vi "ERR HANDLER - Processor Loop.vi"   [LabVIEW 2013]
uses:
  Error Queue Message.ctl
types:
  T1 = typedef "Error Queue Message.ctl" = cluster{"Command":enum16{"HANDLE ERROR", "EXIT"}, "Data":variant}
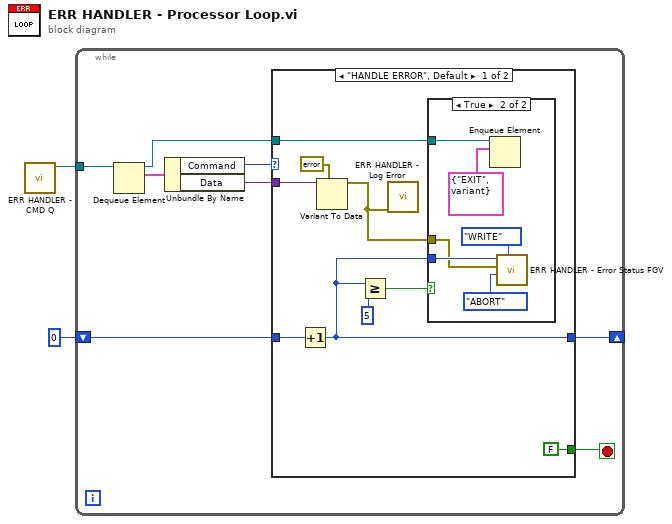
[diagram p0: block diagram]
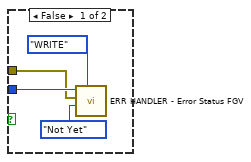
[diagram p2: hidden frame]
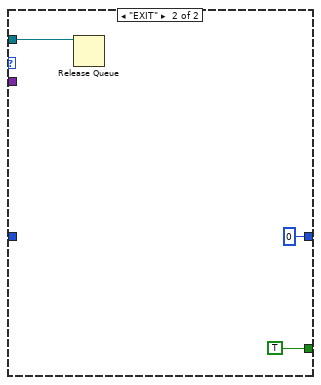
[diagram p3: hidden frame]
diagram:
  n1 = call "ERR HANDLER - CMD Q.vi"() -> ("Err Handler Q"=w2:refnum<queue>)  [unwired: 11 in]
  n2 = while {
    tunnel: w2 -> [w10]
    shift-right: [w3] -> _
    shift-left: 0 -> [w4]
    stop <- w7 stop-if-true
    n3 = Dequeue Element(queue=w10) -> (queue out=w6:refnum<queue>, element=w9:T1)  [unwired: 2 in, 2 out]
    n4 = Unbundle By Name(w9) -> ("Command"=w8:enum16{"HANDLE ERROR", "EXIT"}, "Data"=w5:variant)
    n5 = case shown="\"HANDLE ERROR\", Default" w8 {
      tunnel: [FALSE TRUE] -> w7
      tunnel: w6 -> [w13 w31]
      tunnel: w5 -> [w19 _]
      tunnel: w4 -> [w16 _]
      tunnel: [w12 0] -> w3
      frame "HANDLE ERROR", Default {
        n6 = Increment(x=w16) -> (x+1=w12:i32)
        n7 = Variant To Data(type=errorcluster {"status"=FALSE, "code"=0, "source"=""} ("error constant"), Variant=w19) -> (data=w11:errorcluster)  [unwired: 1 in, 1 out]
        n8 = Greater Or Equal?(x=w12, y=5) -> (x >= y?=w14:bool)
        n9 = call "ERR HANDLER - Log Error.vi"("error"=w11) -> ()  [unwired: 10 in, 1 out]
        n10 = case shown="True" w14 {
          tunnel: w13 -> [_ w29]
          tunnel: w12 -> [w22 w27]
          tunnel: w11 -> [w21 w26]
          frame False {
            n11 = call "ERR HANDLER - Error Status FGV.vi"("Method"=enum16{"READ", "WRITE"}."WRITE", "Abort Program (W)"=enum16{"Not Yet", "ABORT"}."Not Yet", "Last Error (W)"=w21, "Error Count (W)"=w22) -> ()  [unwired: 5 in, 3 out]
          }
          frame True {
            n12 = Enqueue Element(queue=w29, element=T1 {"Command"=enum."EXIT", "Data"=variant} ("Error Handler Mesg")) -> ()  [unwired: 2 in, 3 out]
            n13 = call "ERR HANDLER - Error Status FGV.vi"("Method"=enum16{"READ", "WRITE"}."WRITE", "Abort Program (W)"=enum16{"Not Yet", "ABORT"}."ABORT", "Last Error (W)"=w26, "Error Count (W)"=w27) -> ()  [unwired: 5 in, 3 out]
          }
        }
      }
      frame "EXIT" {
        n14 = Release Queue(queue=w31) -> ()  [unwired: 2 in, 3 out]
      }
    }
  }
